vi "[ToBeTest] N-Parametric Double FFT Mesurament RT.vi"() -> ()   [LabVIEW 2014]
uses:
  <vilib>/Platform/TimedLoop/XDataNode/timing_clust.ctl
  <vilib>/Platform/TimedLoop/XDataNode/nitl_modes.ctl
  <vilib>/Platform/TimedLoop/XDataNode/wakeup.ctl
  <vilib>/FPGAPlugInAG/sbRIO-9636/niLvFpga_Open_sbRIO-9636.vi
  <vilib>/rvi/interface/common/dynamic/niFpgaDynamicAddResources.vi
  <vilib>/FPGAPlugInAG/Dynamic/niLvFpga_Reset_Dynamic.vi
  <vilib>/Utility/error.llb/Error Cluster From Error Code.vi
  <vilib>/rvi/errors/niLvFpgaAdjustHostInterfaceError.vi
  <vilib>/rvi/interface/common/niFpgaWaitOnOcc.vi
  <vilib>/FPGAPlugInAG/Dynamic/niLvFpga_Run_Dynamic.vi
  <vilib>/FPGAPlugInAG/Dynamic/niLvFpga_Abort_Dynamic.vi
  <vilib>/FPGAPlugInAG/Dynamic/niLvFpga_Close_Dynamic.vi
  <vilib>/rvi/interface/nirviOpenFPGA/nirviOpenFPGA.xnode
  FPGA Bitfiles/LaserDistanceSen_FPGATarget_N-ParametricDoub_YVLbjAYtdP4.lvbitx
  FPGA Target/Test VIs/N-Parametric Double FFT Mesurament Test.vi
  <vilib>/rvi/interface/nirviMethod/nirviMethod.xnode
  <vilib>/rvi/interface/nirviReadWriteControl/nirviReadWriteControl.xnode
  <vilib>/platform/TimedLoop/XDataNode/XDataNode.xnode
  <vilib>/rvi/interface/nirviCloseFPGA/nirviCloseFPGA.xnode
  <vilib>/FPGAPlugInAG/Dynamic/niLvFpga_ConfigureFifo_Dynamic.vi
  <vilib>/rvi/errors/niLvFpgaMergeErrorWithErrorCode.vi
  <vilib>/FPGAPlugInAG/Dynamic/niLvFpga_StartFifo_Dynamic.vi
  <vilib>/rvi/interface/Simulation/niFpgaSimulationCallBeginRW.vi
  <vilib>/FPGAPlugInAG/Dynamic/niLvFpga_ReadFifo_Dynamic.vi
  <vilib>/Platform/TimedLoop/XDataNode/XDNodeRunTimeDep.lvlib
  NiFpgaLv.dll
panel:
  in  "tieni premuto per":i32=1
  out "Second Std Deviations %":dbl[](array[numeric])
  out "First Std Deviations %":dbl[](array[numeric])
  out "Second Mean Freq Curves":dbl[][](graph)
  out "First Mean Freq Curves":dbl[][](graph)
  in  "# Measurements for Linearization":i32=10
  out "Current Signal":i32
  in  "Linearization?":bool
  in  "Triangular Multiply Factor":dbl[](array[numeric])=[1.0, 0.95, 0.9, 0.85, 0.8]
  out "Second Edge N-FFT":dbl[](graph)
  in  "Enable triangular scaling":bool
  in  "Triangolo dritto?":bool=TRUE
  out "First Edge N-FFT":dbl[](graph)
  in  "#Signals":u32(slide)=5 scale=1.0..5.0
  in  "stop":bool
  in  "Initial Latency points":u32(slide) scale=0.0..1249.0
  out "Elements Remaining FFT":u32
  out "Elements Remaining Signal":u32
  out "N-Signals":dbl[](graph)
  in  "Snapshot":bool
  in  "Windowing":T1(ring)
  in  "first bin":i32=5
  in  "last bin":i32=255
  in  "lower limit 2":u32(slide)=738 scale=625.0..738.0
  in  "lower limit 1":u32(slide)=113 scale=0.0..113.0
  # "WARNING:\nOnce pressed wait untill the end of operation"
  # "OFFLINE parameters"
  # "Max Detection FFT bin range"
  # "ONLINE parameters"
  # "1st triangular"
  # "2nd triangular"
  # "3rd triangular"
  # "4th triangular"
  # "5th triangular"
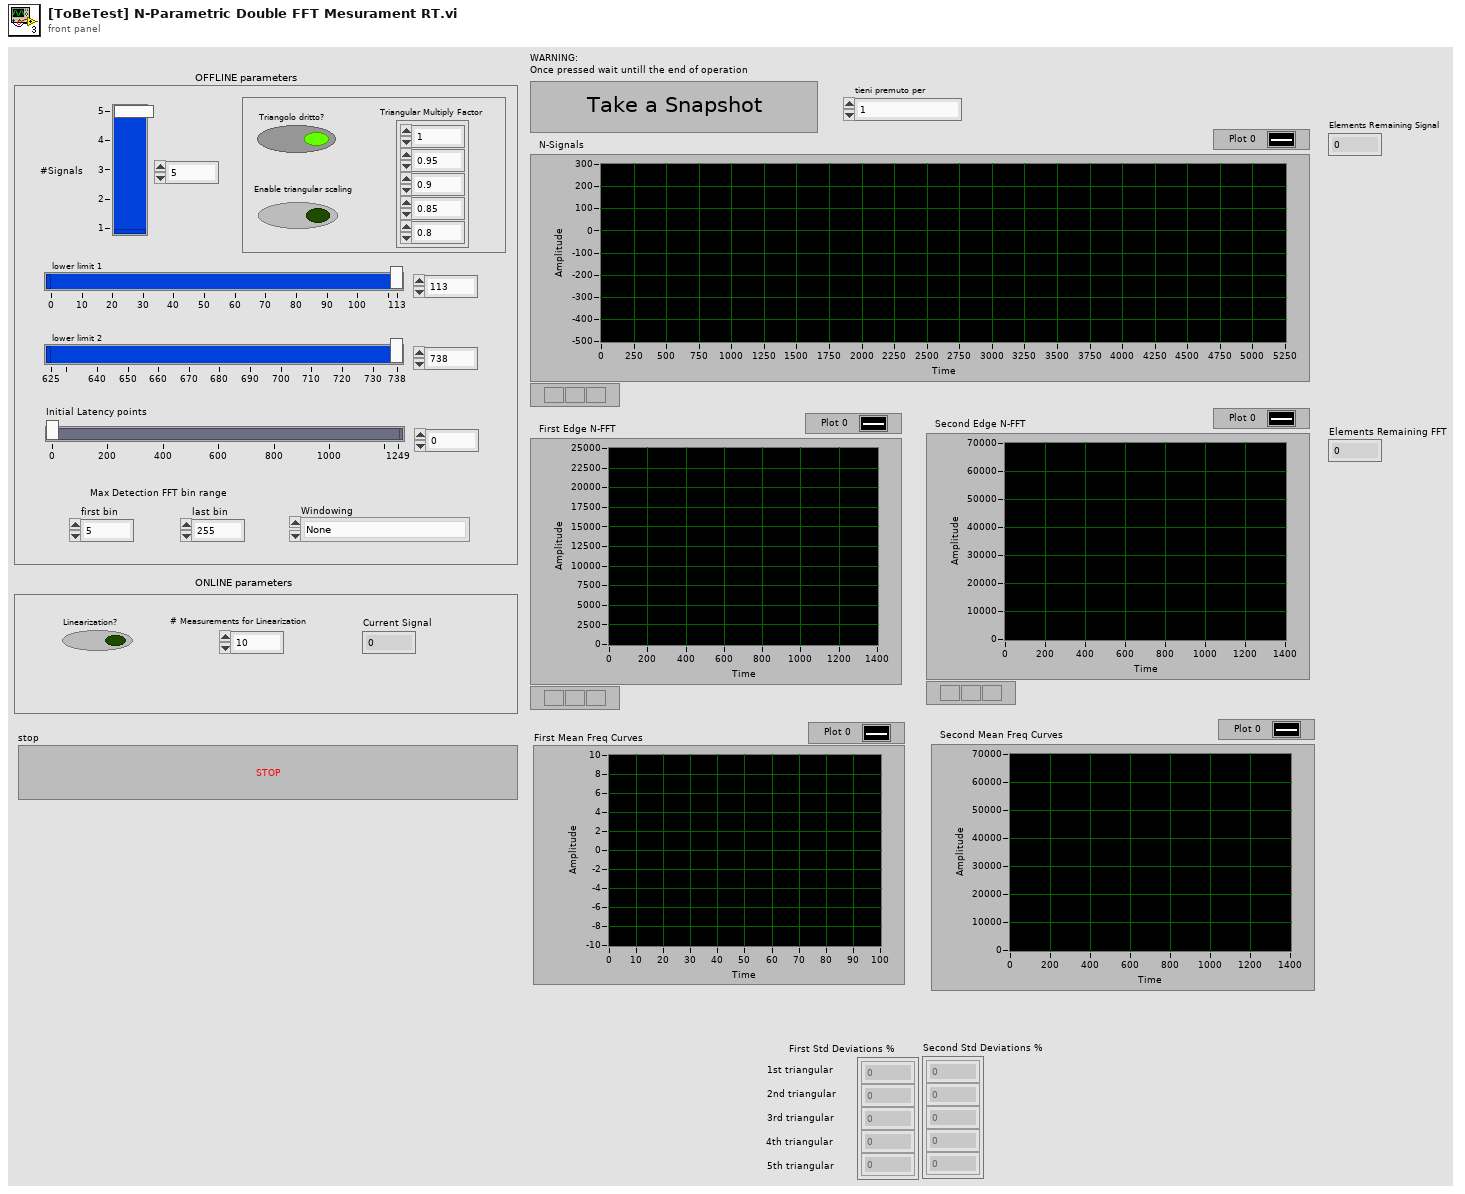
[diagram p1: front panel]
types:
  T1 = enum16{"None", "Hanning", "Hamming", "Blackman", "Blackman-Harris"}
  T2 = typedef "XDNodeRunTimeDep.lvlib/timing_clust.ctl" = cluster{"Expected End [f-1]":u64, "Actual End [f-1]":u64, "Finished Late? [f-1]":bool, "Expected End [i-1]":u64, "Actual End [i-1]":u64, "Finished Late? [i-1]":bool, "Expected Start [i]":u64, "Actual Start [i]":u64, "Expected Start [f]":u64, "Actual Start [f]":u64, "Source Name":string, "Structure Name":string, "Period":i64, "Deadline":i64, "Offset":i64, "Start":i64, "Priority":i32, "Timeout":i32, "Mode":T3, "Wakeup Reason":T4, "Error":errorcluster, "Source Type":string, "Secondary Source Type":string, "Global End Time":u64, "Global Start Time":u64, "Frame Duration":u64, "Iteration Duration":u64, "Assigned CPU":i32, "I/O Scan Engine Mode":u32}
  T3 = typedef "XDNodeRunTimeDep.lvlib/nitl_modes.ctl" = enum32{"No Change", "Process missed periods, maintain original phase", "Discard missed periods, maintain original phase", "Process missed periods, ignore original phase", "Discard missed periods, ignore original phase"}
  T4 = typedef "XDNodeRunTimeDep.lvlib/wakeup.ctl" = enum32{"Normal", "Aborted", "Asynchronous wakeup", "Timing source error", "Timed loop error", "Timeout"}
  T5 = typedef "NI_Matrix.lvlib/RealMatrix.ctl" = dbl[][]
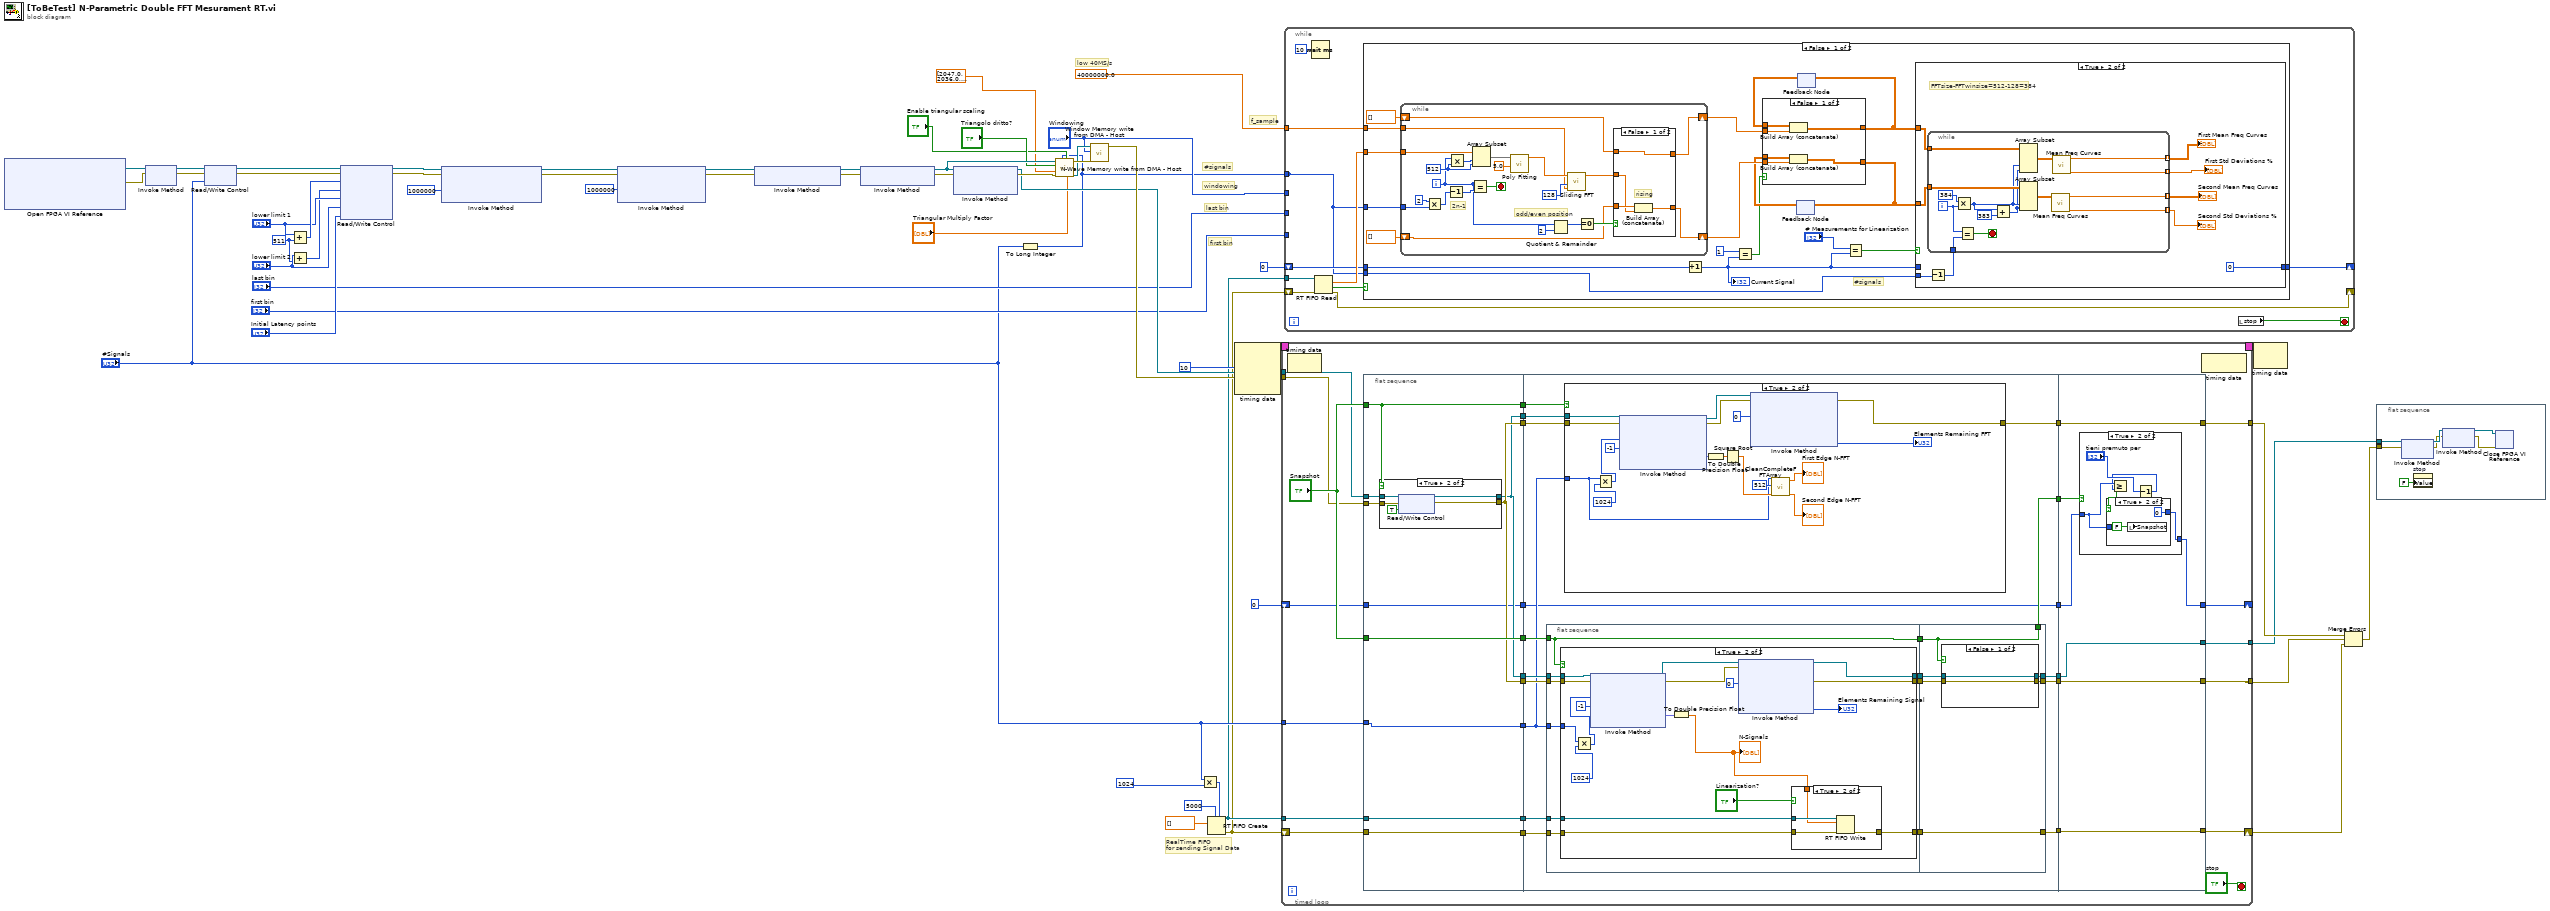
[diagram p0: block diagram]
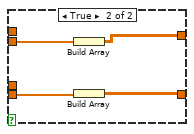
[diagram p3: hidden frame]
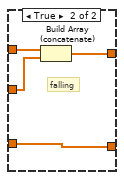
[diagram p4: hidden frame]
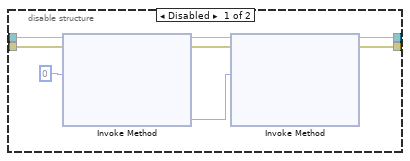
[diagram p8: hidden frame]
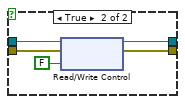
[diagram p10: hidden frame]
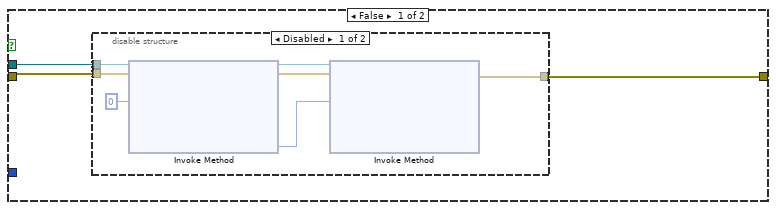
[diagram p11: hidden frame]
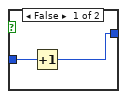
[diagram p14: hidden frame]
diagram:
  w51 = u32 511 ("y")
  # "f_sample"
  # "#signals"
  # "RealTime FIFO \nfor sending Signal Data"
  # "windowing"
  # "last bin"
  # "first bin"
  # "low 40MS/s"
  n1 = xnode "Open FPGA VI Reference"() -> ("FPGA VI Reference Out"=w25:refnum<k20>, "error out"=w24:errorcluster)  [unwired: 2 in]
  n2 = xnode "Invoke Method"("FPGA VI Reference In"=w25, "error in"=w24) -> ("FPGA VI Reference Out"=w22:refnum<k20>, "error out"=w23:errorcluster)
  n3 = xnode "Read/Write Control"("FPGA VI Reference In"=w22, "error in"=w23, "n"="#Signals") -> ("FPGA VI Reference Out"=w21:refnum<k20>, "error out"=w20:errorcluster)
  n4 = Add(x="lower limit 1", y=w51) -> (x+y=w55:u32)
  n5 = Add(x="lower limit 2", y=w51) -> (x+y=w53:u32)
  n6 = xnode "Read/Write Control"("FPGA VI Reference In"=w21, "error in"=w20, "upper limit 1"=w55, "upper limit 2"=w53, "lower limit 1"="lower limit 1", "lower limit 2"="lower limit 2", "Latency points"="Initial Latency points") -> ("FPGA VI Reference Out"=w49:refnum<k20>, "error out"=w48:errorcluster)
  n7 = xnode "Invoke Method"("FPGA VI Reference In"=w49, "error in"=w48, "Requested Depth"=u32 1000000) -> ("FPGA VI Reference Out"=w36:refnum<k20>, "error out"=w37:errorcluster)  [unwired: 1 out]
  n8 = xnode "Invoke Method"("FPGA VI Reference In"=w36, "error in"=w37, "Requested Depth"=u32 1000000) -> ("FPGA VI Reference Out"=w43:refnum<k20>, "error out"=w44:errorcluster)  [unwired: 1 out]
  n9 = xnode "Invoke Method"("FPGA VI Reference In"=w43, "error in"=w44) -> ("FPGA VI Reference Out"=w34:refnum<k20>, "error out"=w35:errorcluster)
  n10 = xnode "Invoke Method"("FPGA VI Reference In"=w34, "error in"=w35) -> ("FPGA VI Reference Out"=w29:refnum<k20>, "error out"=w42:errorcluster)
  n11 = xnode "Invoke Method"("FPGA VI Reference In"=w29, "error in"=w42) -> ("FPGA VI Reference Out"=w30:refnum<k20>, "error out"=w33:errorcluster)  [unwired: 1 in]
  n12 = To Long Integer(number="#Signals") -> (32bit integer=w4:i32)
  n13 = call "N-Wave Memory write from DMA - Host.vi"("Triangular Multiply Factor"="Triangular Multiply Factor", "Enable triangular scaling"="Enable triangular scaling", "n"=w4, "error in"=w33, "Custom Triangular Signal (fal-ris)"=dbl[] [2047.0, 2036.0, 2024.0, 2013.0, 2002.0, 1990.0, 1979.0, 1968.0, 1956.0, 1945.0, 1934.0, 1923.0, 1912.0, 1900.0, 1889.0, 1878.0, 1867.0, 1856.0, 1845.0, 1833.0, 1822.0, 1811.0, 1800.0, 1789.0, 1778.0, 1767.0, 1756.0, 1745.0, 1734.0, 1723.0, 1712.0, 1702.0, 1691.0, 1680.0, 1669.0, 1658.0, 1647.0, 1636.0, 1626.0, 1615.0, 1604.0, 1593.0, 1583.0, 1572.0, 1561.0, 1550.0, 1540.0, 1529.0, 1518.0, 1508.0, 1497.0, 1487.0, 1476.0, 1465.0, 1455.0, 1444.0, 1434.0, 1423.0, 1413.0, 1402.0, 1392.0, 1381.0, 1371.0, 1360.0, 1350.0, 1340.0, 1329.0, 1319.0, 1309.0, 1298.0, 1288.0, 1278.0, 1267.0, 1257.0, 1247.0, 1237.0, 1226.0, 1216.0, 1206.0, 1196.0, 1186.0, 1176.0, 1165.0, 1155.0, 1145.0, 1135.0, 1125.0, 1115.0, 1105.0, 1095.0, 1085.0, 1075.0, 1065.0, 1055.0, 1045.0, 1035.0, 1025.0, 1015.0, 1006.0, 996.0, 986.0, 976.0, 966.0, 956.0, 947.0, 937.0, 927.0, 917.0, 908.0, 898.0, 888.0, 879.0, 869.0, 859.0, 850.0, 837.0, 826.0, 816.0, 804.0, 796.0, 788.0, 778.0, 769.0, 758.0, 750.0, 743.0, 733.0, 724.0, 717.0, 709.0, 701.0, 693.0, 686.0, 677.0, 669.0, 661.0, 653.0, 645.0, 638.0, 630.0, 622.0, 615.0, 607.0, 599.0, 592.0, 583.0, 576.0, 569.0, 561.0, 554.0, 547.0, 539.0, 532.0, 525.0, 518.0, 509.0, 501.0, 492.0, 486.0, 478.0, 471.0, 463.0, 456.0, 450.0, 442.0, 435.0, 429.0, 421.0, 415.0, 408.0, 401.0, 394.0, 388.0, 381.0, 375.0, 368.0, 361.0, 355.0, 349.0, 342.0, 336.0, 330.0, 323.0, 317.0, 311.0, 304.0, 298.0, 292.0, 286.0, 279.0, 273.0, 267.0, 261.0, 255.0, 249.0, 242.0, 236.0, 230.0, 224.0, 218.0, 212.0, 206.0, 200.0, 194.0, 187.0, 181.0, 175.0, 169.0, 163.0, 157.0, 150.0, 144.0, 138.0, 132.0, 125.0, 119.0, 113.0, 107.0, 101.0, 95.0, 88.0, 82.0, 77.0, 71.0, 65.0, 59.0, 53.0, 47.0, 41.0, 35.0, 29.0, 23.0, 18.0, 11.0, 6.0, 0.0, -6.0, -12.0, -18.0, -23.0, -29.0, -35.0, -41.0, -47.0, -52.0, -58.0, -64.0, -69.0, -75.0, -81.0, -87.0, -92.0, -98.0, -104.0, -109.0, -115.0, -121.0, -126.0, -132.0, -138.0, -144.0, -149.0, -155.0, -161.0, -166.0, -172.0, -177.0, -183.0, -189.0, -194.0, -200.0, -205.0, -211.0, -216.0, -222.0, -227.0, -233.0, -238.0, -244.0, -249.0, -255.0, -260.0, -266.0, -271.0, -277.0, -283.0, -288.0, -294.0, -299.0, -304.0, -310.0, -315.0, -321.0, -326.0, -331.0, -337.0, -342.0, -348.0, -353.0, -358.0, -364.0, -369.0, -375.0, -380.0, -385.0, -391.0, -396.0, -402.0, -407.0, -413.0, -418.0, -423.0, -429.0, -434.0, -439.0, -445.0, -450.0, -456.0, -461.0, -466.0, -472.0, -477.0, -483.0, -488.0, -493.0, -499.0, -504.0, -510.0, -515.0, -520.0, -526.0, -531.0, -537.0, -542.0, -548.0, -553.0, -558.0, -564.0, -569.0, -574.0, -580.0, -585.0, -590.0, -596.0, -601.0, -606.0, -612.0, -617.0, -622.0, -628.0, -633.0, -638.0, -644.0, -649.0, -654.0, -660.0, -665.0, -670.0, -676.0, -681.0, -686.0, -692.0, -697.0, -702.0, -708.0, -713.0, -718.0, -723.0, -729.0, -734.0, -739.0, -744.0, -750.0, -755.0, -760.0, -765.0, -771.0, -776.0, -781.0, -786.0, -792.0, -797.0, -802.0, -807.0, -812.0, -818.0, -823.0, -828.0, -833.0, -839.0, -844.0, -849.0, -854.0, -859.0, -865.0, -870.0, -875.0, -880.0, -885.0, -891.0, -896.0, -901.0, -906.0, -911.0, -916.0, -922.0, -927.0, -932.0, -937.0, -943.0, -948.0, -953.0, -958.0, -963.0, -969.0, -974.0, -979.0, -984.0, -989.0, -995.0, -1000.0, -1005.0, -1010.0, -1015.0, -1021.0, -1026.0, -1031.0, -1036.0, -1041.0, -1047.0, -1052.0, -1057.0, -1062.0, -1067.0, -1073.0, -1078.0, -1083.0, -1088.0, -1093.0, -1099.0, -1104.0, -1109.0, -1114.0, -1119.0, -1124.0, -1130.0, -1135.0, -1140.0, -1145.0, -1150.0, -1156.0, -1161.0, -1166.0, -1171.0, -1176.0, -1182.0, -1187.0, -1192.0, -1197.0, -1202.0, -1207.0, -1213.0, -1218.0, -1223.0, -1228.0, -1233.0, -1238.0, -1244.0, -1249.0, -1254.0, -1259.0, -1264.0, -1269.0, -1275.0, -1280.0, -1285.0, -1290.0, -1295.0, -1300.0, -1305.0, -1311.0, -1316.0, -1321.0, -1326.0, -1331.0, -1336.0, -1342.0, -1347.0, -1352.0, -1357.0, -1362.0, -1367.0, -1372.0, -1378.0, -1383.0, -1388.0, -1393.0, -1398.0, -1403.0, -1408.0, -1414.0, -1419.0, -1424.0, -1429.0, -1434.0, -1439.0, -1444.0, -1450.0, -1455.0, -1460.0, -1465.0, -1470.0, -1475.0, -1480.0, -1486.0, -1491.0, -1496.0, -1501.0, -1506.0, -1511.0, -1516.0, -1522.0, -1527.0, -1532.0, -1537.0, -1542.0, -1547.0, -1552.0, -1558.0, -1563.0, -1568.0, -1573.0, -1578.0, -1583.0, -1588.0, -1593.0, -1599.0, -1604.0, -1609.0, -1614.0, -1619.0, -1624.0, -1629.0, -1634.0, -1640.0, -1645.0, -1650.0, -1655.0, -1660.0, -1665.0, -1670.0, -1675.0, -1681.0, -1686.0, -1691.0, -1696.0, -1701.0, -1706.0, -1711.0, -1716.0, -1722.0, -1727.0, -1732.0, -1737.0, -1742.0, -1747.0, -1752.0, -1757.0, -1762.0, -1768.0, -1773.0, -1778.0, -1783.0, -1788.0, -1793.0, -1798.0, -1803.0, -1808.0, -1814.0, -1819.0, -1824.0, -1829.0, -1834.0, -1839.0, -1844.0, -1849.0, -1854.0, -1859.0, -1865.0, -1870.0, -1875.0, -1880.0, -1885.0, -1890.0, -1895.0, -1900.0, -1905.0, -1911.0, -1916.0, -1921.0, -1926.0, -1931.0, -1936.0, -1941.0, -1946.0, -1951.0, -1956.0, -1961.0, -1967.0, -1972.0, -1977.0, -1982.0, -1987.0, -1992.0, -1997.0, -2002.0, -2007.0, -2012.0, -2017.0, -2023.0, -2028.0, -2033.0, -2038.0, -2043.0, -2048.0, -2047.0, -2034.0, -2021.0, -2009.0, -1996.0, -1983.0, -1970.0, -1957.0, -1945.0, -1932.0, -1919.0, -1907.0, -1894.0, -1881.0, -1869.0, -1856.0, -1844.0, -1831.0, -1819.0, -1806.0, -1794.0, -1781.0, -1769.0, -1757.0, -1744.0, -1732.0, -1719.0, -1707.0, -1695.0, -1682.0, -1670.0, -1658.0, -1646.0, -1634.0, -1621.0, -1609.0, -1597.0, -1585.0, -1573.0, -1561.0, -1549.0, -1537.0, -1525.0, -1513.0, -1501.0, -1489.0, -1477.0, -1465.0, -1453.0, -1441.0, -1429.0, -1417.0, -1405.0, -1394.0, -1382.0, -1370.0, -1358.0, -1347.0, -1335.0, -1323.0, -1312.0, -1300.0, -1288.0, -1277.0, -1265.0, -1254.0, -1242.0, -1231.0, -1219.0, -1208.0, -1196.0, -1185.0, -1173.0, -1162.0, -1150.0, -1139.0, -1128.0, -1116.0, -1105.0, -1094.0, -1083.0, -1071.0, -1060.0, -1049.0, -1038.0, -1027.0, -1015.0, -1004.0, -993.0, -982.0, -971.0, -960.0, -949.0, -938.0, -927.0, -916.0, -905.0, -894.0, -883.0, -873.0, -862.0, -851.0, -840.0, -829.0, -819.0, -808.0, -797.0, -786.0, -776.0, -765.0, -754.0, -744.0, -733.0, -722.0, -712.0, -697.0, -685.0, -674.0, -661.0, -652.0, -643.0, -632.0, -622.0, -610.0, -602.0, -594.0, -583.0, -574.0, -566.0, -558.0, -550.0, -542.0, -534.0, -525.0, -516.0, -507.0, -499.0, -491.0, -483.0, -475.0, -467.0, -459.0, -451.0, -443.0, -435.0, -426.0, -419.0, -411.0, -404.0, -396.0, -388.0, -381.0, -373.0, -366.0, -359.0, -349.0, -341.0, -331.0, -325.0, -317.0, -309.0, -301.0, -295.0, -288.0, -280.0, -273.0, -266.0, -259.0, -252.0, -246.0, -239.0, -231.0, -225.0, -219.0, -212.0, -205.0, -199.0, -192.0, -186.0, -180.0, -173.0, -167.0, -161.0, -155.0, -148.0, -142.0, -136.0, -130.0, -124.0, -118.0, -112.0, -106.0, -100.0, -94.0, -88.0, -82.0, -76.0, -70.0, -64.0, -58.0, -52.0, -46.0, -40.0, -34.0, -28.0, -21.0, -15.0, -9.0, -3.0, 2.0, 9.0, 15.0, 21.0, 27.0, 33.0, 39.0, 45.0, 51.0, 57.0, 63.0, 69.0, 75.0, 81.0, 86.0, 92.0, 98.0, 103.0, 110.0, 116.0, 121.0, 127.0, 133.0, 138.0, 144.0, 149.0, 155.0, 161.0, 166.0, 172.0, 177.0, 183.0, 189.0, 194.0, 200.0, 205.0, 211.0, 216.0, 221.0, 227.0, 232.0, 238.0, 243.0, 249.0, 254.0, 259.0, 265.0, 270.0, 276.0, 281.0, 286.0, 292.0, 297.0, 303.0, 308.0, 314.0, 319.0, 324.0, 329.0, 335.0, 340.0, 345.0, 351.0, 356.0, 361.0, 366.0, 371.0, 377.0, 382.0, 387.0, 392.0, 397.0, 403.0, 408.0, 413.0, 418.0, 423.0, 429.0, 434.0, 439.0, 444.0, 449.0, 454.0, 459.0, 464.0, 469.0, 474.0, 479.0, 484.0, 489.0, 494.0, 499.0, 504.0, 509.0, 514.0, 520.0, 525.0, 530.0, 535.0, 540.0, 545.0, 550.0, 555.0, 560.0, 565.0, 570.0, 575.0, 580.0, 585.0, 590.0, 595.0, 600.0, 605.0, 610.0, 615.0, 620.0, 625.0, 630.0, 636.0, 641.0, 646.0, 651.0, 656.0, 661.0, 666.0, 671.0, 676.0, 681.0, 686.0, 691.0, 696.0, 701.0, 706.0, 711.0, 716.0, 721.0, 726.0, 731.0, 736.0, 741.0, 746.0, 751.0, 756.0, 761.0, 765.0, 770.0, 775.0, 780.0, 785.0, 790.0, 795.0, 800.0, 805.0, 810.0, 815.0, 820.0, 825.0, 829.0, 834.0, 839.0, 844.0, 849.0, 854.0, 859.0, 864.0, 868.0, 873.0, 878.0, 883.0, 888.0, 893.0, 897.0, 902.0, 907.0, 912.0, 917.0, 921.0, 926.0, 931.0, 936.0, 941.0, 945.0, 950.0, 955.0, 960.0, 965.0, 969.0, 974.0, 979.0, 984.0, 988.0, 993.0, 998.0, 1003.0, 1007.0, 1012.0, 1017.0, 1022.0, 1027.0, 1031.0, 1036.0, 1041.0, 1046.0, 1051.0, 1055.0, 1060.0, 1065.0, 1070.0, 1075.0, 1079.0, 1084.0, 1089.0, 1094.0, 1098.0, 1103.0, 1108.0, 1113.0, 1118.0, 1122.0, 1127.0, 1132.0, 1137.0, 1141.0, 1146.0, 1151.0, 1156.0, 1161.0, 1165.0, 1170.0, 1175.0, 1180.0, 1184.0, 1189.0, 1194.0, 1199.0, 1204.0, 1208.0, 1213.0, 1218.0, 1223.0, 1227.0, 1232.0, 1237.0, 1242.0, 1246.0, 1251.0, 1256.0, 1261.0, 1265.0, 1270.0, 1275.0, 1280.0, 1284.0, 1289.0, 1294.0, 1299.0, 1303.0, 1308.0, 1313.0, 1318.0, 1322.0, 1327.0, 1332.0, 1336.0, 1341.0, 1346.0, 1351.0, 1355.0, 1360.0, 1365.0, 1370.0, 1374.0, 1379.0, 1384.0, 1388.0, 1393.0, 1398.0, 1403.0, 1407.0, 1412.0, 1417.0, 1421.0, 1426.0, 1431.0, 1436.0, 1440.0, 1445.0, 1450.0, 1454.0, 1459.0, 1464.0, 1469.0, 1473.0, 1478.0, 1483.0, 1487.0, 1492.0, 1497.0, 1502.0, 1506.0, 1511.0, 1516.0, 1520.0, 1525.0, 1530.0, 1535.0, 1539.0, 1544.0, 1549.0, 1553.0, 1558.0, 1563.0, 1567.0, 1572.0, 1577.0, 1582.0, 1586.0, 1591.0, 1596.0, 1600.0, 1605.0, 1610.0, 1614.0, 1619.0, 1624.0, 1628.0, 1633.0, 1638.0, 1643.0, 1647.0, 1652.0, 1657.0, 1661.0, 1666.0, 1671.0, 1675.0, 1680.0, 1685.0, 1689.0, 1694.0, 1699.0, 1703.0, 1708.0, 1713.0, 1717.0, 1722.0, 1727.0, 1731.0, 1736.0, 1741.0, 1746.0, 1750.0, 1755.0, 1760.0, 1764.0, 1769.0, 1774.0, 1778.0, 1783.0, 1788.0, 1792.0, 1797.0, 1802.0, 1806.0, 1811.0, 1816.0, 1820.0, 1825.0, 1830.0, 1834.0, 1839.0, 1844.0, 1848.0, 1853.0, 1858.0, 1862.0, 1867.0, 1871.0, 1876.0, 1881.0, 1885.0, 1890.0, 1895.0, 1899.0, 1904.0, 1909.0, 1913.0, 1918.0, 1923.0, 1927.0, 1932.0, 1937.0, 1941.0, 1946.0, 1951.0, 1955.0, 1960.0, 1965.0, 1969.0, 1974.0, 1978.0, 1983.0, 1988.0, 1992.0, 1997.0, 2002.0, 2006.0, 2011.0, 2016.0, 2020.0, 2025.0, 2029.0, 2034.0, 2039.0, 2043.0, 2048.0] ("Complete SkewTri"), "Triangolo dritto?"="Triangolo dritto?", "FPGA VI Reference In"=w29) -> ("FPGA VI Reference Out"=w31:refnum<k20>, "error out"=w32:errorcluster)  [unwired: 2 in, 1 out]
  n14 = call "Window Memory write from DMA - Host.vi"("error in"=w32, "Enum"="Windowing", "FPGA VI Reference In"=w31) -> ("error out"=w50:errorcluster)  [unwired: 5 in, 3 out]
  n15 = Multiply(x="#Signals", y=u32 1024 ("elements in array (1)")) -> (x*y=w10:u32)
  n16 = RT FIFO Create(1:dbl[] [] ("double precision float"), 4:u32 5000 ("size (10)"), 6:w10) -> (8:w6:refnum<k33>, 11:w5:errorcluster)  [unwired: 5 in, 1 out]
  n17 = node-c288(i64 10 ("Period")) -> (w28:T2)  [unwired: 3 in]
  n18 = timed-loop {
    tunnel: w30 -> [w80]
    tunnel: w50 -> [w81]
    tunnel: [w83] -> w41
    tunnel: [w84] -> w40
    tunnel: [w69] -> w38
    tunnel: "#Signals" -> [w66]
    timing: w28 -> [_]
    timing-out: [_] -> w27
    tunnel: w6 -> [w64]
    shift-right: [w60] -> w7
    shift-left: w5 -> [w62]
    shift-right: [w56] -> _
    shift-left: 0 -> [w59]
    stop <- "stop" stop-if-true
    n19 = node-c288() -> ()  [unwired: 1 in, 1 out]
    n20 = flat-sequence {
      tunnel: w80 -> [w93]
      tunnel: w81 -> [w94]
      tunnel: "Snapshot" -> [w91]
      tunnel: "Snapshot" -> [w96]
      tunnel: [w95] -> w79
      tunnel: [w96] -> w78
      tunnel: [w91] -> w77
      tunnel: [w95] -> w76
      tunnel: [w92] -> w75
      tunnel: [w92] -> w74
      tunnel: [w90] -> w67
      tunnel: w66 -> [w90]
      tunnel: [w89] -> w65
      tunnel: w64 -> [w89]
      tunnel: [w88] -> w63
      tunnel: w62 -> [w88]
      tunnel: w59 -> [w87]
      tunnel: [w87] -> w58
      tunnel: w79 -> [w118]
      tunnel: w78 -> [w112]
      tunnel: w77 -> [w115]
      tunnel: w76 -> [w114]
      tunnel: w75 -> [w113]
      tunnel: w74 -> [w119]
      tunnel: [w117] -> w73
      tunnel: [w116] -> w72
      tunnel: [w111] -> w71
      tunnel: [w110] -> w68
      tunnel: w67 -> [w109]
      tunnel: w65 -> [w108]
      tunnel: w63 -> [w107]
      tunnel: [w106] -> w61
      tunnel: w58 -> [w104]
      tunnel: [w104] -> w57
      tunnel: [w216] -> w83
      tunnel: [w217] -> w84
      tunnel: w73 -> [w217]
      tunnel: w72 -> [w216]
      tunnel: w71 -> [w213]
      tunnel: [w215] -> w69
      tunnel: w68 -> [w215]
      tunnel: w61 -> [w214]
      tunnel: [w214] -> w60
      tunnel: w57 -> [w212]
      tunnel: [w211] -> w56
      frame #0 {
        n21 = case shown="True" w91 {
          tunnel: [w97 w103] -> w95
          tunnel: w94 -> [w97 w102]
          tunnel: w93 -> [w98 w101]
          tunnel: [w98 w100] -> w92
          frame False {
          }
          frame True {
            n22 = xnode "Read/Write Control"("FPGA VI Reference In"=w101, "error in"=w102, "snapshot"=TRUE) -> ("FPGA VI Reference Out"=w100:refnum<k20>, "error out"=w103:errorcluster)
          }
        }
      }
      frame #1 {
        n23 = flat-sequence {
          tunnel: w119 -> [w131]
          tunnel: w118 -> [w130]
          tunnel: w112 -> [w127]
          tunnel: [w129] -> w122
          tunnel: [w128] -> w121
          tunnel: [w127] -> w120
          tunnel: w109 -> [w126]
          tunnel: w108 -> [w125]
          tunnel: w107 -> [w124]
          tunnel: [w123] -> w105
          tunnel: [w173] -> w116
          tunnel: w122 -> [w175]
          tunnel: w121 -> [w174]
          tunnel: w120 -> [w172]
          tunnel: [w172] -> w111
          tunnel: [w171] -> w110
          tunnel: [w170] -> w106
          tunnel: w105 -> [w170]
          frame #0 {
            n24 = case shown="True" w127 {
              tunnel: w131 -> [w136 w164]
              tunnel: w130 -> [w135 w163]
              tunnel: [w134 w162] -> w128
              tunnel: [w133 w161] -> w129
              tunnel: w126 -> [_ w160]
              tunnel: w125 -> [_ w151]
              tunnel: w124 -> [w132 w150]
              tunnel: [w132 w149] -> w123
              frame False {
                n25 = disable-structure shown="Enabled" {
                  disable-tunnel: w136 -> [w143 w146]
                  disable-tunnel: w135 -> [w141 w145]
                  disable-tunnel: [w140 w145] -> w134
                  disable-tunnel: [w137 w146] -> w133
                  frame Disabled {
                    n26 = xnode "Invoke Method"("FPGA VI Reference In"=w143, "error in"=w141, "Number of Elements"=u32 0) -> ("FPGA VI Reference Out"=w139:refnum<k20>, "error out"=w138:errorcluster, "Elements Remaining"=w142:u32)  [unwired: 1 in, 1 out]
                    n27 = xnode "Invoke Method"("FPGA VI Reference In"=w139, "error in"=w138, "Number of Elements"=w142) -> ("FPGA VI Reference Out"=w137:refnum<k20>, "error out"=w140:errorcluster)  [unwired: 1 in, 2 out]
                  }
                  frame Enabled {
                  }
                }
              }
              frame True {
                n28 = Multiply(x=w160, y=u32 1024 ("Number of Elements")) -> (x*y=w154:u32)
                n29 = xnode "Invoke Method"("FPGA VI Reference In"=w164, "error in"=w163, "Number of Elements"=w154, "Timeout (ms)"=-1) -> ("FPGA VI Reference Out"=w157:refnum<k20>, "error out"=w156:errorcluster, "Data"=w159:fxp<+/-,12,12>[])  [unwired: 1 out]
                n30 = To Double Precision Float(number=w159) -> (double precision float=w147:dbl[])
                "N-Signals" <- w147
                n31 = xnode "Invoke Method"("FPGA VI Reference In"=w157, "error in"=w156, "Number of Elements"=u32 0) -> ("FPGA VI Reference Out"=w161:refnum<k20>, "error out"=w162:errorcluster, "Elements Remaining"=→"Elements Remaining Signal":u32)  [unwired: 1 in, 1 out]
                n32 = case shown="True" "Linearization?" {
                  tunnel: w151 -> [_ w169]
                  tunnel: w150 -> [w165 w168]
                  tunnel: [w165 w167] -> w149
                  tunnel: w147 -> [_ w166]
                  frame False {
                  }
                  frame True {
                    n33 = RT FIFO Write(0:w169, 1:w166, 3:w168) -> (11:w167:errorcluster)  [unwired: 2 in, 3 out]
                  }
                }
              }
            }
          }
          frame #1 {
            n34 = case shown="False" w172 {
              tunnel: [w177 w180] -> w173
              tunnel: w175 -> [w176 w181]
              tunnel: w174 -> [w177 w179]
              tunnel: [w176 w178] -> w171
              frame False {
              }
              frame True {
                n35 = xnode "Read/Write Control"("FPGA VI Reference In"=w181, "error in"=w179, "snapshot"=FALSE) -> ("FPGA VI Reference Out"=w178:refnum<k20>, "error out"=w180:errorcluster)
              }
            }
          }
        }
        n36 = case shown="True" w115 {
          tunnel: w113 -> [w185 w209]
          tunnel: w114 -> [w184 w210]
          tunnel: [w183 w208] -> w117
          tunnel: w109 -> [_ w194]
          frame False {
            n37 = disable-structure shown="Disabled" {
              disable-tunnel: w185 -> [w191 _]
              disable-tunnel: w184 -> [w188 w193]
              disable-tunnel: [w187 w193] -> w183
              frame Disabled {
                n38 = xnode "Invoke Method"("FPGA VI Reference In"=w191, "error in"=w188, "Number of Elements"=u32 0) -> ("FPGA VI Reference Out"=w189:refnum<k20>, "error out"=w186:errorcluster, "Elements Remaining"=w190:u32)  [unwired: 1 in, 1 out]
                n39 = xnode "Invoke Method"("FPGA VI Reference In"=w189, "error in"=w186, "Number of Elements"=w190) -> ("error out"=w187:errorcluster)  [unwired: 1 in, 3 out]
              }
              frame Enabled {
              }
            }
          }
          frame True {
            n40 = Multiply(x=w194, y=u32 1024 ("Number of Elements")) -> (x*y=w200:u32)
            n41 = xnode "Invoke Method"("FPGA VI Reference In"=w209, "error in"=w210, "Number of Elements"=w200, "Timeout (ms)"=-1) -> ("FPGA VI Reference Out"=w204:refnum<k20>, "error out"=w205:errorcluster, "Data"=w207:fxp<+,44,44>[])  [unwired: 1 out]
            n42 = To Double Precision Float(number=w207) -> (double precision float=w206:dbl[])
            n43 = Square Root(x=w206) -> (sqrt(x)=w197:dbl[])
            n44 = xnode "Invoke Method"("FPGA VI Reference In"=w204, "error in"=w205, "Number of Elements"=u32 0) -> ("error out"=w208:errorcluster, "Elements Remaining"=→"Elements Remaining FFT":u32)  [unwired: 1 in, 2 out]
            n45 = call "CleanCompleteFFTArray.vi"("Complete FFT Array"=w197, "FFT Size"=512, "#Signals"=w194) -> ("Second Edge Array"=→"Second Edge N-FFT":dbl[], "First Edge Array"=→"First Edge N-FFT":dbl[])  [unwired: 7 in]
          }
        }
      }
      frame #2 {
        n46 = case shown="True" w213 {
          tunnel: w212 -> [w218 w222]
          tunnel: [w218 w223] -> w211
          frame False {
          }
          frame True {
            n47 = Decrement(x="tieni premuto per") -> (x-1=w219:i32)
            n48 = Greater Or Equal?(x=w222, y=w219) -> (x >= y?=w221:bool)
            n49 = case shown="True" w221 {
              tunnel: w222 -> [w224 _]
              tunnel: [w225 0] -> w223
              frame False {
                n50 = Increment(x=w224) -> (x+1=w225:i32)
              }
              frame True {
                n51 = local write "Snapshot"(FALSE ("Snapshot")) -> ()
              }
            }
          }
        }
      }
    }
    n52 = node-c288() -> ()  [unwired: 1 in, 1 out]
  }
  n53 = while {
    tunnel: "first bin" -> [_]
    tunnel: "last bin" -> [_]
    tunnel: "Windowing" -> [_]
    tunnel: w6 -> [w238]
    shift-right: [w232] -> _
    shift-left: w5 -> [w237]
    tunnel: [w229] -> _
    tunnel: w4 -> [w229]
    tunnel: 40000000.0 ("Sample Rate (S/s)") -> [w233]
    shift-right: [w230] -> _
    shift-left: 0 ("first bin") -> [w231]
    stop <- w228 stop-if-true
    n54 = Wait (ms)(milliseconds to wait=u32 10 ("millisecond multiple")) -> ()  [unwired: 1 out]
    n55 = RT FIFO Read(0:w238, 3:w237) -> (9:w234:dbl[], 10:w236:bool, 11:w232:errorcluster)  [unwired: 2 in, 2 out]
    n56 = case shown="False" w236 {
      tunnel: w234 -> [w257 _]
      tunnel: w229 -> [w256 _]
      tunnel: w233 -> [w255 _]
      tunnel: w231 -> [w248 w323]
      tunnel: [w242 w323] -> w230
      tunnel: w229 -> [w239 _]
      frame False {
        # "#signals"
        n57 = while {
          tunnel: w257 -> [w314]
          shift-right: [w294] -> w252
          shift-left: dbl[] [] ("SubtractedSignal") -> [w297]
          tunnel: w256 -> [w309]
          tunnel: w255 -> [w302]
          shift-right: [w293] -> w251
          shift-left: dbl[] [] ("SubtractedSignal") -> [w296]
          i -> [w301]
          stop <- w305 stop-if-true
          w312 = 512 ("y")
          # "odd/even position"
          # "2n-1"
          n58 = Multiply(x=2, y=w309) -> (x*y=w307:i32)
          n59 = Decrement(x=w307) -> (x-1=w306:i32)
          n60 = Multiply(x=w301, y=w312) -> (x*y=w313:i32)
          n61 = Equal?(x=w301, y=w306) -> (x = y?=w305:bool)
          n62 = Array Subset(array=w314, index=w313, length=w312) -> (w311:dbl[])
          n63 = call "Poly Fitting.vi"("Poly Grade"=5.0, "Signal"=w311) -> ("SubtractedSignal"=w303:dbl[])  [unwired: 8 in, 1 out]
          n64 = Quotient & Remainder(x=w301, y=2) -> (x-y*floor(x/y)=w299:i32)  [unwired: 1 out]
          n65 = call "Sliding FFT.vi"("Sample Freq"=w302, "FFT Win Size"=128, "SubSmoothSignal"=w303) -> ("Freq samples"=w295:dbl[])  [unwired: 7 in, 1 out]
          n66 = Equal To 0?(x=w299) -> (x = 0?=w298:bool)
          n67 = case shown="False" w298 {
            tunnel: w297 -> [w316 w321]
            tunnel: w296 -> [w318 w319]
            tunnel: w295 -> [w317 w322]
            tunnel: [w316 w320] -> w294
            tunnel: [w315 w319] -> w293
            frame False {
              # "rising"
              n68 = Build Array (concatenate)(w318, w317) -> (w315:dbl[])
            }
            frame True {
              # "falling"
              n69 = Build Array (concatenate)(w321, w322) -> (w320:dbl[])
            }
          }
        }
        n70 = Increment(x=w248) -> (x+1=w244:i32)
        "Current Signal" <- w244
        n71 = Equal?(x=1, y=w244) -> (x = y?=w246:bool)
        n72 = feedback #1() -> (w249:T5)  [unwired: 1 in]
        n73 = feedback #2() -> (w250:T5)  [unwired: 1 in]
        n74 = case shown="False" w246 {
          tunnel: w251 -> [w287 w290]
          tunnel: w252 -> [w288 w292]
          tunnel: [w286 w289] -> w241
          tunnel: [w285 w291] -> w240
          tunnel: w250 -> [w284 _]
          tunnel: w249 -> [w283 _]
          frame False {
            n75 = Build Array (concatenate)(w284, w288) -> (w285:T5)
            n76 = Build Array (concatenate)(w283, w287) -> (w286:T5)
          }
          frame True {
            n77 = Build Array(w292) -> (w291:T5)
            n78 = Build Array(w290) -> (w289:T5)
          }
        }
        n79 = feedback-in #1(w241) -> ()
        n80 = feedback-in #2(w240) -> ()
        n81 = Equal?(x="# Measurements for Linearization", y=w244) -> (x = y?=w243:bool)
        n82 = case shown="True" w243 {
          tunnel: w244 -> [w258 _]
          tunnel: [w258 0] -> w242
          tunnel: w241 -> [_ w265]
          tunnel: w240 -> [_ w266]
          tunnel: w239 -> [_ w264]
          frame False {
          }
          frame True {
            # "FFTsize-FFTwinsize=512-128=384"
            n83 = Decrement(x=w264) -> (x-1=w263:i32)
            n84 = while {
              tunnel: w266 -> [w282]
              tunnel: w265 -> [w281]
              tunnel: w263 -> [w275]
              tunnel: [w271] -> w259 mode=indexing
              tunnel: [w270] -> w260 mode=indexing
              tunnel: [w269] -> w261 mode=indexing
              tunnel: [w268] -> w262 mode=indexing
              i -> [w276]
              stop <- w274 stop-if-true
              n85 = Multiply(x=384 ("# Measurements for Linearization 2"), y=w276) -> (x*y=w279:i32)
              n86 = Equal?(x=w276, y=w275) -> (x = y?=w274:bool)
              n87 = Add(x=w279, y=383) -> (x+y=w277:i32)
              n88 = Array Subset(array=w282, index (col)=w279, length (col)=w277) -> (w273:T5)  [unwired: 2 in]
              n89 = Array Subset(array=w281, index (col)=w279, length (col)=w277) -> (w272:T5)  [unwired: 2 in]
              n90 = call "Mean Freq Curves.vi"("Set of Freq samples"=w272) -> ("StdDev%"=w271:dbl, "Mean Freq Curve"=w269:dbl[])  [unwired: 9 in]
              n91 = call "Mean Freq Curves.vi"("Set of Freq samples"=w273) -> ("StdDev%"=w270:dbl, "Mean Freq Curve"=w268:dbl[])  [unwired: 9 in]
            }
            "First Mean Freq Curves" <- w262
            "Second Mean Freq Curves" <- w261
            "First Std Deviations %" <- w260
            "Second Std Deviations %" <- w259
          }
        }
      }
      frame True {
      }
    }
    n92 = local read "stop"() -> (w228:bool)
  }
  n93 = node-c288(w27) -> ()  [unwired: 1 out]
  n94 = Merge Errors(w40, w41, w7) -> (w45:errorcluster)
  n95 = flat-sequence {
    tunnel: w45 -> [w330]
    tunnel: w38 -> [w325]
    frame #0 {
      n96 = xnode "Invoke Method"("FPGA VI Reference In"=w325, "error in"=w330) -> ("FPGA VI Reference Out"=w327:refnum<k20>, "error out"=w326:errorcluster)
      n97 = property on="stop" class="Bool (strict)"("Value"=FALSE ("stop")) -> ()  [unwired: 2 in, 2 out]
      n98 = xnode "Invoke Method"("FPGA VI Reference In"=w327, "error in"=w326) -> ("FPGA VI Reference Out"=w328:refnum<k20>, "error out"=w329:errorcluster)
      n99 = xnode "Close FPGA VI Reference"("FPGA VI Reference In"=w328, "error in"=w329) -> ()  [unwired: 1 out]
    }
  }
